vi "countToAngle.vi"(8 "error in (no error)":errorcluster, 10 "Encoder 1 Count":u32, 11 "Encoder 0 Count":u32) -> (0 "error out":errorcluster, 2 "Enc 1 angle (rad)":dbl, 3 "Enc 0 angle (rad)":dbl)   [LabVIEW 2017, in "externalAquisition.lvlib"]
doc: "This VI converts the encoder counts to angles in radians."
uses:
  externalAquisition.lvlib
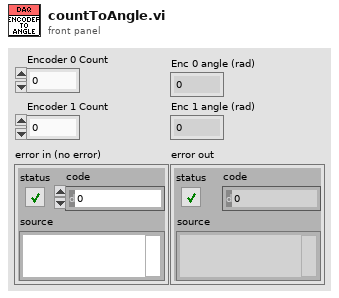
[diagram p1: front panel]
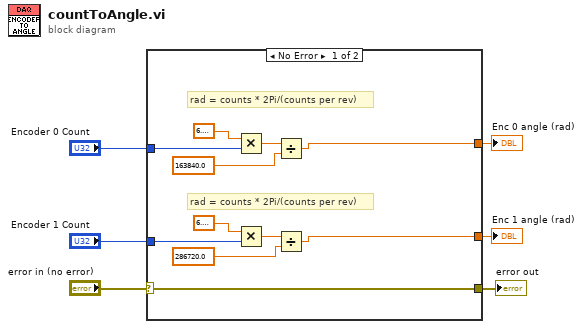
[diagram p0: block diagram]
diagram:
  n1 = case shown="No Error" "error in (no error)" {
    selector: "error in (no error)" -> [w13 w18]
    tunnel: [w13 w18] -> w5
    tunnel: "Encoder 0 Count" -> [w16 _]
    tunnel: "Encoder 1 Count" -> [w14 _]
    tunnel: [w10 _] -> w2
    tunnel: [w9 _] -> w1
    frame No Error {
      # "rad = counts * 2Pi/(counts per rev)"
      # "rad = counts * 2Pi/(counts per rev)"
      n2 = Multiply(x=6.283185307179586, y=w16) -> (x*y=w12:dbl)
      n3 = Multiply(x=6.283185307179586, y=w14) -> (x*y=w11:dbl)
      n4 = Divide(x=w12, y=163840.0) -> (x/y=w10:dbl)
      n5 = Divide(x=w11, y=286720.0) -> (x/y=w9:dbl)
    }
    frame Error {
    }
  }
  "error out" <- w5
  "Enc 0 angle (rad)" <- w2
  "Enc 1 angle (rad)" <- w1
